vi "GT Home Stop.vi"(6 "acc":dbl, 7 "vel":dbl, 8 "error in (no error)":errorcluster caption="错误输入（无错误）", 9 "pos":i32, 10 "axis":i16, 11 "cardNum":i16) -> (0 "error out":errorcluster caption="错误输出", 3 "function return":i16)   [LabVIEW 2020, in "gts.lvlib"]
doc: "GT_API GT_HomeStop(short cardNum,short axis,long pos,double vel,double acc);"
uses:
  gts.lvlib
  dll/32bit/multi_card/gts.dll
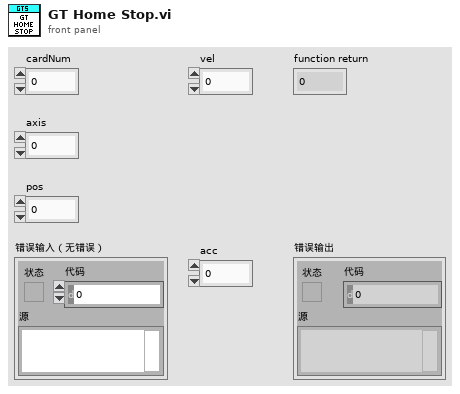
[diagram p1: front panel]
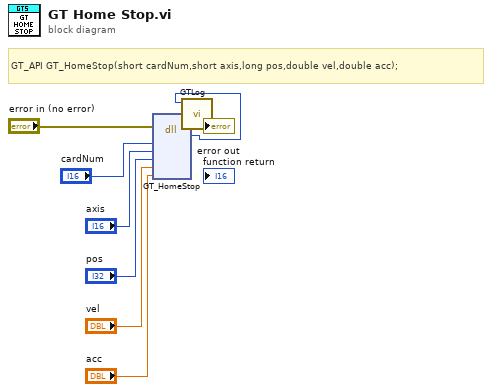
[diagram p0: block diagram]
diagram:
  # "GT_API GT_HomeStop(short cardNum,short axis,long pos,double vel,double acc);"
  n1 = dll-call lib="C:/1228/dll/32bit/multi_card/gts.dll" fn="GT_HomeStop"(error in="error in (no error)", "cardNum"="cardNum", "axis"="axis", "pos"="pos", "vel"="vel", "acc"="acc") -> (error out=w3:errorcluster, w1:i16)  [unwired: 7 in, 1 out]
  n2 = call "GTLog.vi"("error in (no error)"=w3, "Numeric"=w1) -> ("error out"=→"error out":errorcluster)  [unwired: 9 in]
